vi "p186.vi"() -> ()   [LabVIEW 2017]
panel:
  in  "Boolean":bool
  out "Numeric 3":i32
  out "Numeric 2":i32
  out "Numeric":dbl format="%#_13g"
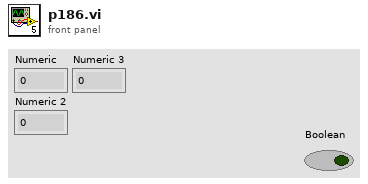
[diagram p1: front panel]
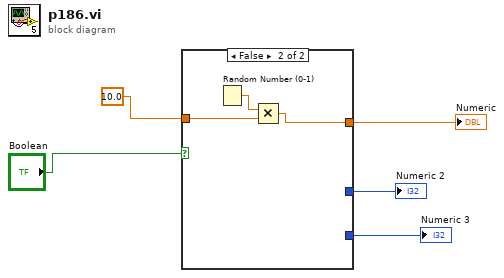
[diagram p0: block diagram]
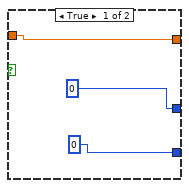
[diagram p2: hidden frame]
diagram:
  n1 = case shown="False" "Boolean" {
    tunnel: 10.0 -> [w8 w10]
    tunnel: [w8 w9] -> w4
    tunnel: [0 _] -> w2
    tunnel: [0 _] -> w1
    frame True {
    }
    frame False {
      n2 = Random Number (0-1)() -> (number: 0 to 1=w11:dbl)
      n3 = Multiply(x=w11, y=w10) -> (x*y=w9:dbl)
    }
  }
  "Numeric" <- w4
  "Numeric 2" <- w2
  "Numeric 3" <- w1
